vi "Patrick-UTiLIA-Sim-SetupAq.vi"(5 "Sampling Info":cluster{"Fs":dbl[unit], "#S":i32}={"Fs"=71808.0, "#S"=16384}, 6 "Ref Phase":dbl=-1.6 format="%.2f", 7 "Ref Frequency":dbl[unit]=1122.0 min=0.0 max=10000.0 step=50.0, 8 "Ref Amplitude":dbl=0.25 min=0.0 max=0.3 step=0.05 format="%.2f") -> (0 "Error out":errorcluster, 1 "Unit Quadrature":dbl[](array[numeric]) format="%.2f", 2 "Unit Reference":dbl[](array[numeric]) format="%.2f", 3 "Scaled Reference":dbl[](array[numeric]) format="%.2f", 4 "DAQ Configuration":cluster{"AO TaskID":u32, "AI  TaskID":u32} {"AI  TaskID" format="%.0x"; "AO TaskID" format="%.0x"})   [LabVIEW 2013]
uses:
  <vilib>/Analysis/NI_AALBase.lvlib
panel:
  out "actual trigger params":T1={"level"=0.0, "hysteresis"=0.0020407331, "delay (sec)"=0.0} {"level" format="%.4f"; "hysteresis" format="%.4f"; "delay (sec)" format="%.4f"}
  out "actual update rate":sgl=71808.0 format="%.2f"
  out "Waveform Graph":dbl[](graph)
  out "Cycles/chunk":dbl=256.0 min=0.0 max=10000.0 step=50.0 format="%.2f"
  out "Buffer Size":i32=131072 max=10000 step=50
  in  "Chunks in Buffer":i32=8 max=200 step=2
  out "Chunks/sec":dbl[unit]=4.3828125 min=0.0 max=10000.0 step=50.0 format="%.2p"
  out "Samp/cycle":dbl=64.0 max=2000.0 step=10.0 format="%.2f"
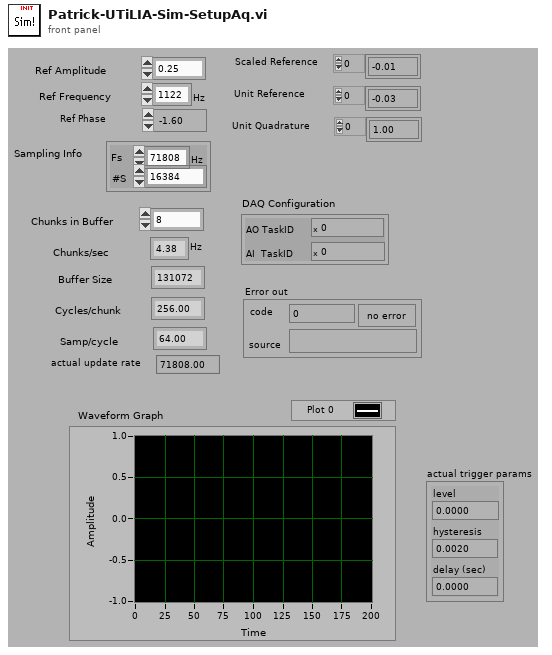
[diagram p1: front panel]
types:
  T1 = cluster{"level":sgl, "hysteresis":sgl, "delay (sec)":sgl}
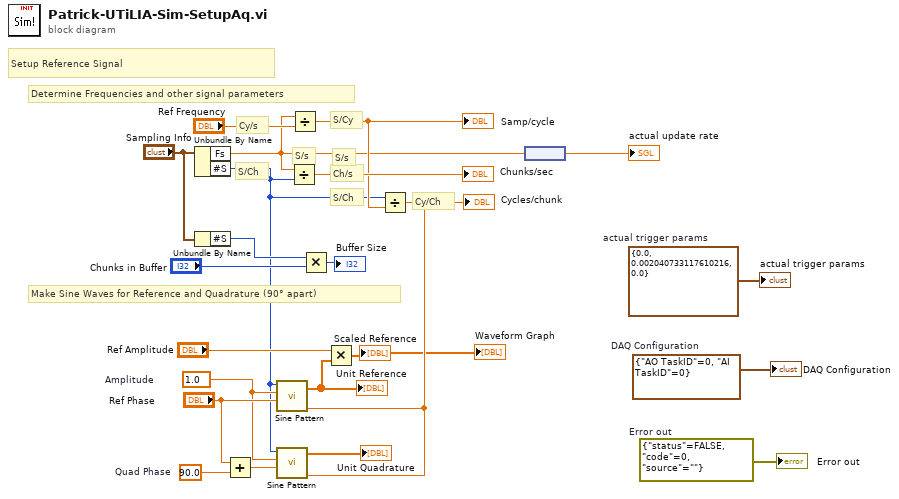
[diagram p0: block diagram]
diagram:
  w1 = T1 {"level"=0.0, "hysteresis"=0.0020407331, "delay (sec)"=0.0}  # actual trigger params
  w5 = cluster{"AO TaskID":u32, "AI  TaskID":u32} {"AO TaskID"=0, "AI  TaskID"=0}  # DAQ Configuration
  w6 = errorcluster {"status"=FALSE, "code"=0, "source"=""}  # Error out
  w17 = 1.0  # Amplitude
  w16 = 90.0  # Quad Phase
  # "Cy/Ch"
  # "S/Ch"
  # "S/s"
  # "Ch/s"
  # "S/Cy"
  # "Cy/s"
  # "S/Ch"
  # "S/s"
  # "Make Sine Waves for Reference and Quadrature (90° apart)"
  # "Determine Frequencies and other signal parameters"
  # "Setup Reference Signal"
  n1 = Unbundle By Name("Sampling Info") -> ("Fs"=w7:dbl[unit], "#S"=w3:i32)
  n2 = Unbundle By Name("Sampling Info") -> ("#S"=w12:i32)
  n3 = Add(x="Ref Phase", y=w16) -> (x+y=w20:dbl)
  n4 = Divide(x=w7, y=w3) -> (x/y=→"Chunks/sec":dbl[unit])
  n5 = Divide(x=w7, y="Ref Frequency") -> (x/y=w9:dbl)
  "Samp/cycle" <- w9
  n6 = Multiply(x=w12, y="Chunks in Buffer") -> (x*y=→"Buffer Size":i32)
  n7 = Divide(x=w3, y=w9) -> (x/y=w10:dbl)
  "Cycles/chunk" <- w10
  n8 = call <vilib>:"Sine Pattern.vi"("cycles"=w10, "phase(degrees)"="Ref Phase", "amplitude"=w17, "samples"=w3) -> ("Sinusoidal Pattern"=w15:dbl[])  [unwired: 1 out]
  "Unit Reference" <- w15
  n9 = call <vilib>:"Sine Pattern.vi"("cycles"=w10, "phase(degrees)"=w20, "amplitude"=w17, "samples"=w3) -> ("Sinusoidal Pattern"=→"Unit Quadrature":dbl[])  [unwired: 1 out]
  n10 = Multiply(x="Ref Amplitude", y=w15) -> (x*y=→"Scaled Reference" →"Waveform Graph":dbl[])
  n11 = node(w7) -> (→"actual update rate":dbl)
  "DAQ Configuration" <- w5
  "Error out" <- w6
  "actual trigger params" <- w1
